vi "GetDBAreaName.vi"(8 "错误输入（无错误）":errorcluster, 11 "ComboBox输入":refnum<vi>) -> (0 "错误输出":errorcluster, 3 "所有记录":string[](array[string]))   [LabVIEW 2014, in "Sample.lvlib"]
uses:
  Sample/Sample.lvlib
  DataBase.lvlib
  DetectElecrodes/DetectElectros.lvlib
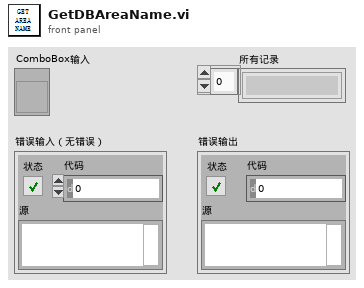
[diagram p1: front panel]
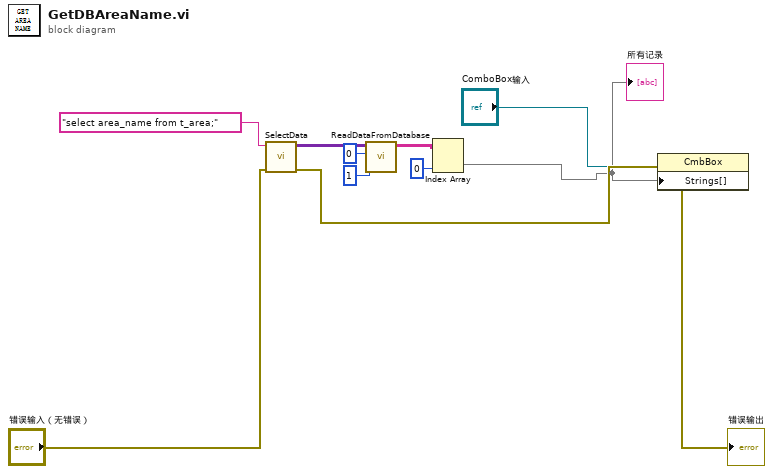
[diagram p0: block diagram]
diagram:
  n1 = call "SelectData.vi"("SQL query"="select area_name from t_area;", "error in"="错误输入（无错误）") -> ("recordset data"=w4:variant[][], "error out"=w9:errorcluster)  [unwired: 6 in]
  n2 = call "ReadDataFromDatabase.vi"("长度"=1, "index"=0, "recordset data"=w4) -> ("所有记录"=w7:string[][])  [unwired: 7 in, 1 out]
  n3 = Index Array(array=w7, index (col)=0 ("禁用的索引 (列)")) -> (element=w1:string[])  [unwired: 1 in]
  "所有记录" <- w1
  n4 = property on="属性节点" class="CmbBox"(reference="ComboBox输入", error in=w9, "Strings[]"=w1) -> (error out=→"错误输出":errorcluster)  [unwired: 1 out]
